vi "catalog.get_dataset.vi"(8 "error in":errorcluster, 10 "Dataset RID":string, 11 "Nominal Client in":refnum<class "Nominal Client.lvclass">) -> (0 "error out":errorcluster, 2 "Dataset":refnum<class "dataset.lvclass">, 3 "Nominal Client out":refnum<class "Nominal Client.lvclass">)   [LabVIEW 2020, in "Nominal Client.lvclass"]
doc: "Retrieve dataset information from RID."
uses:
  Nominal Client.lvclass
  datasources/dataset/dataset.lvclass
  Nominal Client.lvclass/Nominal Client.ctl
  create.authorization_header.vi
  trace.payload_sent.vi
  trace.payload_received.vi
  error.vi
  api_token.get.vi
  trace.calling_method.vi
  <vilib>/JDP Science/JDP Science Common Utilities/Trim Whitespace__JDP.vi
  <vilib>/AdvancedString/1D String Array to Delimited String.vi
  error.vi/859f8e04-e495-489b-b5b4-7ac163f56130.vi
  <vilib>/Utility/libraryn.llb/Get File Extension.vi
  log_file.write.vi
  submodules/reqwest-labview/lv-src/reqwest/get.vi
  <vilib>/JDP Science/JSONtext/Get all Object Items.vi
  <vilib>/Utility/error.llb/Error Cluster From Error Code.vi
  <vilib>/JDP Science/JSONtext/JSON text to Variant.vi
  <vilib>/JDP Science/JSONtext/LVClass Serializer/JSONtext LVClass Serializer.lvclass
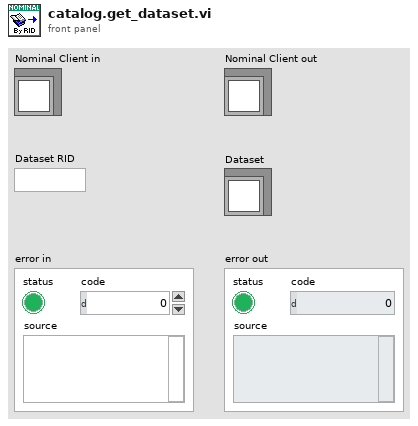
[diagram p1: front panel]
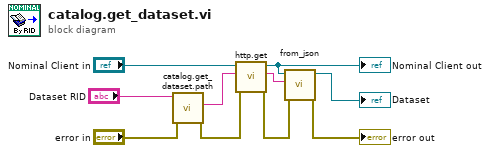
[diagram p0: block diagram]
diagram:
  n1 = call "catalog.get_dataset.path.vi"("error in"="error in", "Dataset UUID"="Dataset RID") -> ("error out"=w8:errorcluster, "path"=w7:string)  [unwired: 8 in]
  n2 = call "http.get.vi"("error in"=w8, "Path"=w7, "Nominal Client in"="Nominal Client in") -> ("error out"=w3:errorcluster, "Response"=w1:string, "Nominal Client out"=w2:refnum<class "Nominal Client.lvclass">)  [unwired: 6 in]
  "Nominal Client out" <- w2
  n3 = call "from_json.vi"("error in"=w3, "dataset JSON"=w1, "Client"=w2) -> ("error out"=→"error out":errorcluster, "Dataset"=→"Dataset":refnum<class "dataset.lvclass">)  [unwired: 7 in]
